vi "AlliGator Load Phasor Ratio References.vi"(8 "Error In":errorcluster, 11 "Reference File Path (default: Dialog)":path) -> (0 "Error Out":errorcluster, 1 "Reference 2 Loaded":bool, 2 "Reference 1 Loaded":bool, 3 "Phasor References":T2, 4 "Message":string)   [LabVIEW 2021, in "AlliGator Phasor Ratio.lvlib"]
doc: "Dialog to select one or both references to load."
uses:
  AlliGator Phasor Ratio.lvlib
  Phasor/Phasor (g, s).ctl
  Phasor Graph/AlliGator Phasor Ratio Reference & Lifetime v1.ctl
  AlliGator Phasor Ratio Reference & Lifetime v2.ctl
  aa7095b5-11c0-4eb5-8147-98e7219ba57f.vi
  aa7095b5-11c0-4eb5-8147-98e7219ba57f.vi/8a80743f-1319-44c8-96b0-3ef8fc688731.vi
  aa7095b5-11c0-4eb5-8147-98e7219ba57f.vi/931f4f8f-d8c6-4056-833f-5c8fe97b24b9.vi
  <vilib>/Utility/error.llb/Error Cluster From Error Code.vi
  <vilib>/ErrorRing/Error Ring.xnode
  Phasor/Phasor.lvlib
  Phasor Graph/AlliGator Phasor Graph.lvlib
  Files/Files.lvlib
  Settings/AlliGator Settings.lvlib
panel:
  in  "Cancel":bool
  in  "Load":bool
  in  "Load Reference 2":bool
  in  "Load Reference 1":bool
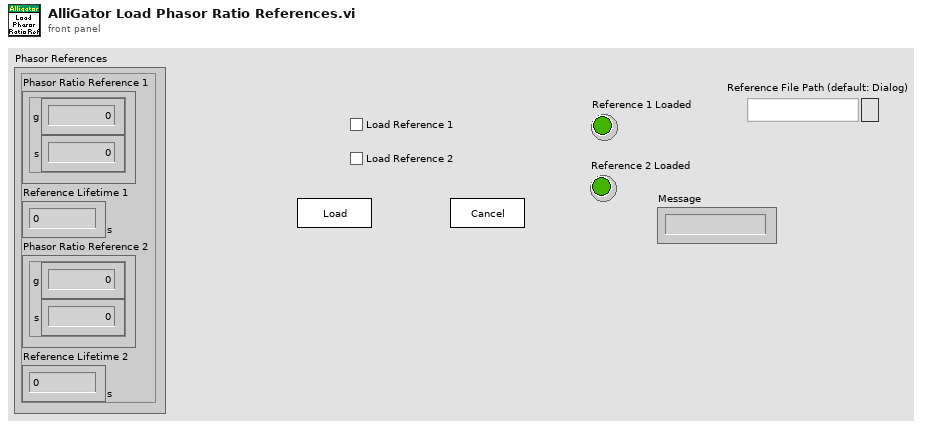
[diagram p1: front panel]
types:
  T1 = typedef "Phasor.lvlib/Phasor (g, s).ctl" = cluster{"g":dbl, "s":dbl}
  T2 = cluster{"Phasor Ratio Reference 1":T1, "Reference Lifetime 1":dbl[unit], "Phasor Ratio Reference 2":T1, "Reference Lifetime 2":dbl[unit]}
  T3 = typedef "AlliGator Phasor Ratio.lvlib/AlliGator Phasor Ratio Reference & Lifetime v2.ctl" = cluster{"Phasor Ratio Reference":T1, "Reference Lifetime":dbl[unit], "Phasor Frequency":dbl[unit]}
  T4 = typedef "AlliGator Phasor Graph.lvlib/AlliGator Phasor Ratio Reference & Lifetime v1.ctl" = cluster{"Phasor Ratio Reference 1":T1, "Reference Lifetime 1":dbl[unit]}
  T5 = enum32{"Invalid", "Standard", "Closed", "Hidden", "Minimized", "Maximized"}
  T6 = enum8{"Enabled", "Disabled", "Disabled and Grayed Out"}
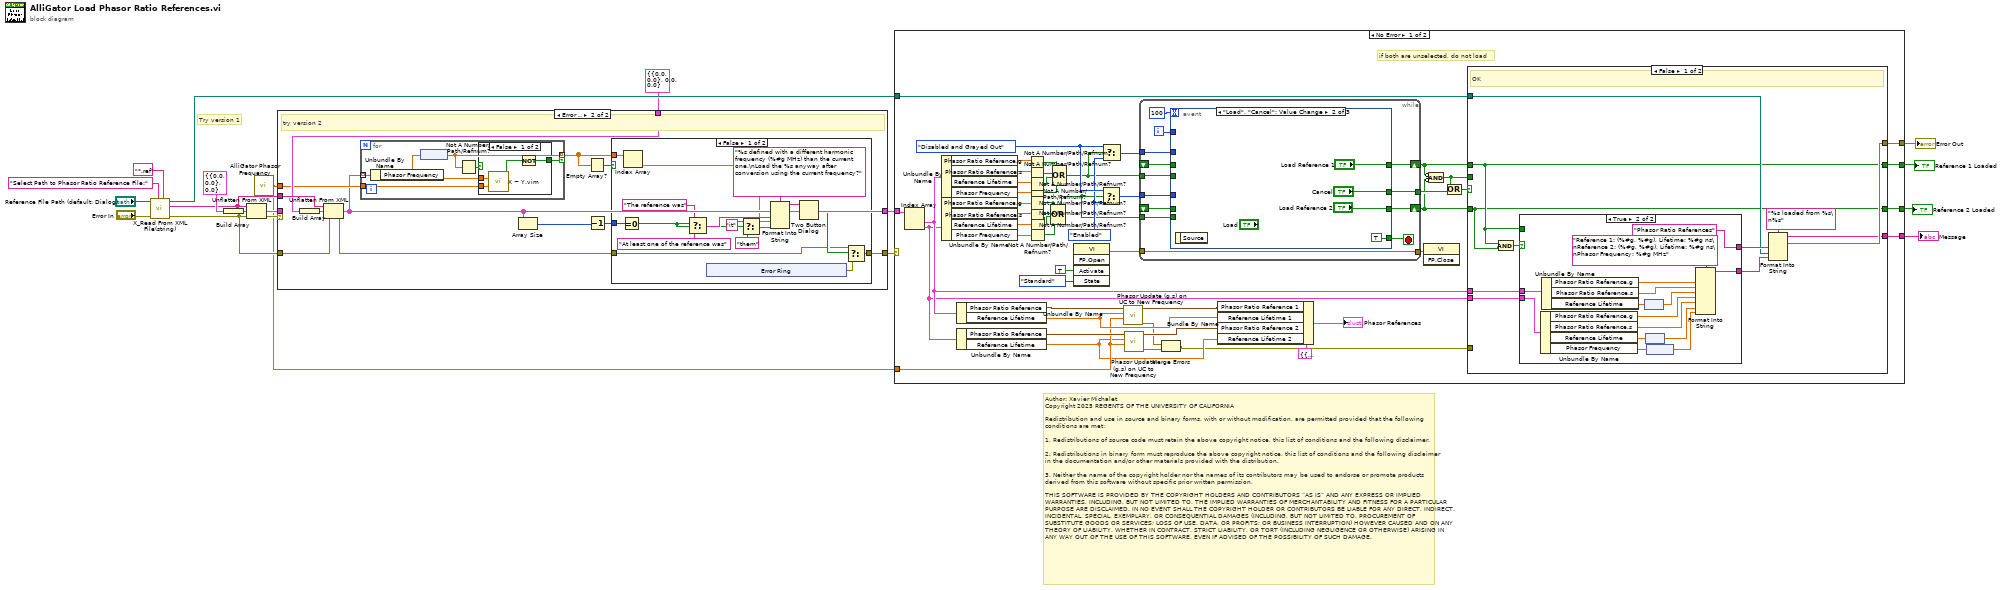
[diagram p0: block diagram]
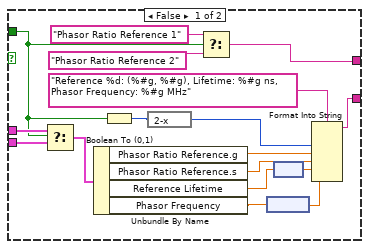
[diagram p2: hidden frame]
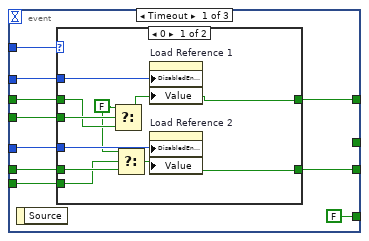
[diagram p4: hidden frame]
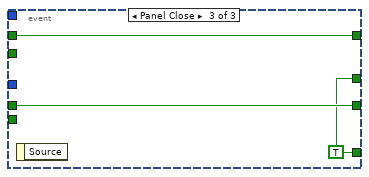
[diagram p6: hidden frame]
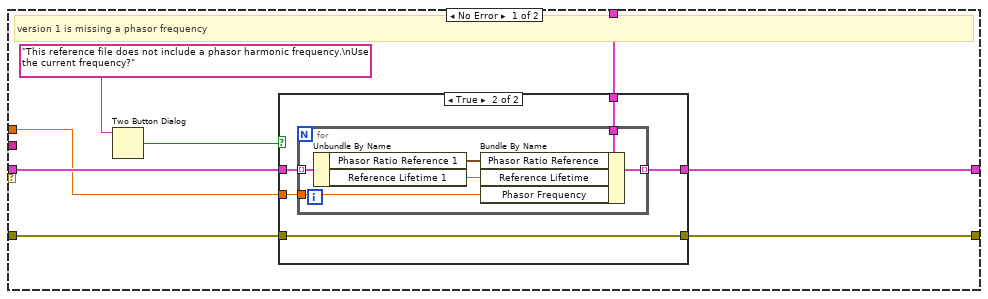
[diagram p8: hidden frame]
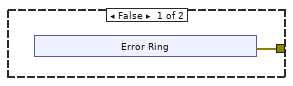
[diagram p9: hidden frame]
diagram:
  # "Author: Xavier Michalet\nCopyright 2025 REGENTS OF THE UNIVERSITY OF CALIFORNIA\n\nRedistribution and use in source and binary forms, with or without modification, are permitted provided that the following conditions are met:\n\n1. Redistributions of source code must retain the above copyright notice, this list of conditions and the following disclaimer.\n\n2. Redistributions in binary form must reproduce the above copyright notice, this list of conditions and the following disclaimer in the documentation and/or other materials provided with the distribution.\n\n3. Neither the name of the copyright holder nor the names of its contributors may be used to endorse or promote products derived from this software without specific prior written permission.\n\nTHIS SOFTWARE IS PROVIDED BY THE COPYRIGHT HOLDERS AND CONTRIBUTORS “AS IS” AND ANY EXPRESS OR IMPLIED WARRANTIES, INCLUDING, BUT NOT LIMITED TO, THE IMPLIED WARRANTIES OF MERCHANTABILITY AND FITNESS FOR A PARTICULAR PURPOSE ARE DISCLAIMED. IN NO EVENT SHALL THE COPYRIGHT HOLDER OR CONTRIBUTORS BE LIABLE FOR ANY DIRECT, INDIRECT, INCIDENTAL, SPECIAL, EXEMPLARY, OR CONSEQUENTIAL DAMAGES (INCLUDING, BUT NOT LIMITED TO, PROCUREMENT OF SUBSTITUTE GOODS OR SERVICES; LOSS OF USE, DATA, OR PROFITS; OR BUSINESS INTERRUPTION) HOWEVER CAUSED AND ON ANY THEORY OF LIABILITY, WHETHER IN CONTRACT, STRICT LIABILITY, OR TORT (INCLUDING NEGLIGENCE OR OTHERWISE) ARISING IN ANY WAY OUT OF THE USE OF THIS SOFTWARE, EVEN IF ADVISED OF THE POSSIBILITY OF SUCH DAMAGE."
  # "Try version 1"
  n1 = call "X_Read From XML File(string).vi"("pattern (*.xml)"="*.ref", "Prompt"="Select Path to Phasor Ratio Reference File:", "error in (no error)"="Error In", "XML File Path"="Reference File Path (default: Dialog)") -> ("error out"=w12:errorcluster, "XML Elements"=w11:string, "XML File Path(duplicate)"=w16:path)  [unwired: 5 in]
  n2 = Build Array(T4 {"Phasor Ratio Reference 1"={"g"=0.0, "s"=0.0}, "Reference Lifetime 1"=0.0} ("appended array")) -> (w7:T4[])
  n3 = Unflatten From XML(xml string=w11, type=w7, error in (no error)=w12) -> (value=w8:T4[], error out=w13:errorcluster)
  n4 = call "AlliGator Phasor Frequency.vi"() -> ("Phasor Frequency"=w1:dbl[unit])
  n5 = case shown="Error .." w13 {
    tunnel: w12 -> [w22 w55]
    tunnel: w11 -> [_ w54]
    tunnel: [w21 w49] -> w6
    tunnel: [w25 w48] -> w10
    tunnel: T3 {"Phasor Ratio Reference"={"g"=0.0, "s"=0.0}, "Reference Lifetime"=0.0, "Phasor Frequency"=0.0} ("appended array") -> [w26 w53]
    tunnel: w8 -> [w27 _]
    tunnel: w1 -> [w20 w51]
    frame No Error {
      # "version 1 is missing a phasor frequency"
      n6 = Two Button Dialog(message="This reference file does not include a phasor harmonic frequency.\nUse the current frequency?") -> (T button?=w23:bool)  [unwired: 2 in]
      n7 = case shown="True" w23 {
        tunnel: w27 -> [_ w37]
        tunnel: w26 -> [_ w36]
        tunnel: [_ w35] -> w25
        tunnel: w22 -> [_ w34]
        tunnel: [w28 w34] -> w21
        tunnel: w20 -> [_ w33]
        frame False {
          n8 = xnode "Error Ring"() -> ("error out"=w28:errorcluster)
        }
        frame True {
          n9 = for {
            tunnel: w37 -> [w43] mode=indexing
            tunnel: w36 -> [w42]
            tunnel: [w39] -> w35 mode=indexing
            tunnel: w33 -> [w38]
            n10 = Unbundle By Name(w43) -> ("Phasor Ratio Reference 1"=w41:T1, "Reference Lifetime 1"=w40:dbl[unit])
            n11 = Bundle By Name(cluster=w42, "Phasor Ratio Reference"=w41, "Reference Lifetime"=w40, "Phasor Frequency"=w38) -> (w39:T3)
          }
        }
      }
    }
    frame Error {
      # "try version 2"
      n12 = Build Array(w53) -> (w52:T3[])
      n13 = Unflatten From XML(xml string=w54, type=w52, error in (no error)=w55) -> (value=w48:T3[], error out=w50:errorcluster)
      n14 = for {
        tunnel: w48 -> [w82] mode=indexing
        tunnel: w51 -> [w81]
        tunnel: [w78] -> w45 mode=indexing if=w80
        n15 = Unbundle By Name(w82) -> ("Phasor Frequency"=w79:dbl[unit])
        n16 = node(w79) -> (w78:dbl)
        n17 = Not A Number/Path/Refnum?(number/path/refnum=w78) -> (NaN/Path/Refnum?=w77:bool)
        n18 = case shown="False" w77 {
          tunnel: w81 -> [w86 _]
          tunnel: [w84 _] -> w80
          tunnel: w79 -> [w83 _]
          frame False {
            n19 = call "X ~ Y.vim"("X"=w83, "Y"=w86) -> ("X ~= Y?"=w85:bool)  [unwired: 13 in]
            n20 = Not(x=w85) -> (.not. x?=w84:bool)
          }
          frame True {
          }
        }
      }
      n21 = Array Size(array=w48) -> (size(s)=w47:i32)
      n22 = Empty Array?(array=w45) -> (empty?=w44:bool)
      n23 = Decrement(x=w47) -> (x-1=w46:i32)
      n24 = case shown="False" w44 {
        tunnel: w50 -> [w58 w76]
        tunnel: [w59 w76] -> w49
        tunnel: w46 -> [w69 _]
        tunnel: w45 -> [w57 _]
        frame False {
          n25 = Equal To 0?(x=w69) -> (x = 0?=w65:bool)
          n26 = Index Array(array=w57) -> (element=w56:dbl)  [unwired: 1 in]
          n27 = Select(t="The reference was" ("message"), s=w65, f="At least one of the reference was" ("message")) -> (s? t:f=w66:string)
          n28 = xnode "Error Ring"() -> ("error out"=w60:errorcluster)
          n29 = Select(t="it" ("message"), s=w65, f="them" ("message")) -> (s? t:f=w62:string)
          n30 = Format Into String(format string="%s defined with a different harmonic frequency (%#g MHz) than the current one.\nLoad the %s anyway after conversion using the current frequency?", w66, w56, w62) -> (resulting string=w71:string)  [unwired: 2 in, 1 out]
          n31 = Two Button Dialog(message=w71) -> (T button?=w61:bool)  [unwired: 2 in]
          n32 = Select(t=w58, s=w61, f=w60) -> (s? t:f=w59:errorcluster)
        }
        frame True {
        }
      }
    }
  }
  n33 = case shown="No Error" w6 {
    selector: w6 -> [_ w222]
    tunnel: [w137 w222] -> w19
    tunnel: w16 -> [w136 _]
    tunnel: [w135 _] -> w15
    tunnel: [w134 _] -> w14
    tunnel: w10 -> [w105 _]
    tunnel: [w99 _] -> w5
    tunnel: w1 -> [w91 _]
    frame No Error {
      w132 = T6."Enabled" ("Disabled")
      w133 = T6."Disabled and Grayed Out" ("Disabled")
      # "if both are unselected, do not load"
      n34 = Index Array(array=w105) -> (element #1=w98:T3, element #2=w97:T3)  [unwired: 2 in]
      n35 = Unbundle By Name(w98) -> ("Phasor Ratio Reference.g"=w116:dbl, "Phasor Ratio Reference.s"=w115:dbl, "Reference Lifetime"=w114:dbl[unit], "Phasor Frequency"=w102:dbl[unit])
      n36 = Unbundle By Name(w97) -> ("Phasor Ratio Reference.g"=w113:dbl, "Phasor Ratio Reference.s"=w112:dbl, "Reference Lifetime"=w111:dbl[unit], "Phasor Frequency"=w104:dbl[unit])
      n37 = Unbundle By Name(w98) -> ("Phasor Ratio Reference"=w96:T1, "Reference Lifetime"=w94:dbl[unit])
      n38 = Unbundle By Name(w97) -> ("Phasor Ratio Reference"=w93:T1, "Reference Lifetime"=w90:dbl[unit])
      n39 = Not A Number/Path/Refnum?(number/path/refnum=w116) -> (NaN/Path/Refnum?=w122:bool)
      n40 = Not A Number/Path/Refnum?(number/path/refnum=w115) -> (NaN/Path/Refnum?=w124:bool)
      n41 = Not A Number/Path/Refnum?(number/path/refnum=w114) -> (NaN/Path/Refnum?=w123:bool)
      n42 = Not A Number/Path/Refnum?(number/path/refnum=w102) -> (NaN/Path/Refnum?=w101:bool)
      n43 = Not A Number/Path/Refnum?(number/path/refnum=w113) -> (NaN/Path/Refnum?=w119:bool)
      n44 = Not A Number/Path/Refnum?(number/path/refnum=w112) -> (NaN/Path/Refnum?=w120:bool)
      n45 = Not A Number/Path/Refnum?(number/path/refnum=w111) -> (NaN/Path/Refnum?=w118:bool)
      n46 = Not A Number/Path/Refnum?(number/path/refnum=w104) -> (NaN/Path/Refnum?=w103:bool)
      n47 = Compound Arithmetic op=OR(w119, w120, w118, w103) -> (w117:bool)
      n48 = Compound Arithmetic op=OR(w122, w124, w123, w101) -> (w121:bool)
      n49 = invoke class="VI" method="FP.Open"("Activate"=TRUE ("Activate?"), "State"=T5."Standard") -> (error out=w106:errorcluster)  [unwired: 3 in, 4 out]
      n50 = Select(t=w133, s=w117, f=w132) -> (s? t:f=w130:T6)
      n51 = Select(t=w133, s=w121, f=w132) -> (s? t:f=w131:T6)
      n52 = call "Phasor Update (g,s) on UC to New Frequency.vi"("New Phasor Frequency"=w91, "Lifetime"=w94, "Phasor in"=w96) -> ("Error Out"=w88:errorcluster, "Phasor out"=w95:T1)  [unwired: 7 in]
      n53 = call "Phasor Update (g,s) on UC to New Frequency.vi"("New Phasor Frequency"=w91, "Lifetime"=w90, "Phasor in"=w93) -> ("Error Out"=w89:errorcluster, "Phasor out"=w92:T1)  [unwired: 7 in]
      n54 = while {
        tunnel: w131 -> [w193]
        tunnel: w130 -> [w192]
        shift-right: [w187] -> w127
        shift-left: _ -> [w190]
        tunnel: w121 -> [w191]
        shift-right: [w186] -> w126
        shift-left: _ -> [w184]
        tunnel: w117 -> [w185]
        tunnel: [w182] -> w129
        tunnel: w106 -> [w181]
        tunnel: [w181] -> w100
        i -> [w188]
        stop <- w183 stop-if-true
        n55 = event shown="[1] \"Load\", \"Cancel\": Value Change" {
          selector: _ -> [_ _ _]
          dyn-events: _ -> [_ _ _]
          timeout: 100 -> [_ _ _]
          tunnel: w193 -> [w203 _ _]
          tunnel: w192 -> [w202 _ _]
          tunnel: w191 -> [w201 _ _]
          tunnel: w190 -> [w200 _ w221]
          tunnel: w188 -> [w199 _ _]
          tunnel: [w198 "Load Reference 1" w221] -> w187
          tunnel: [w197 "Load Reference 2" w220] -> w186
          tunnel: w185 -> [w195 _ _]
          tunnel: w184 -> [w196 _ w220]
          tunnel: [FALSE TRUE w219] -> w183
          tunnel: [_ "Cancel" w219] -> w182
          event Timeout {
            n56 = event-data() -> ()  [unwired: 1 in, 1 out]
            n57 = case shown="0" w199 {
              tunnel: w203 -> [w212 _]
              tunnel: w202 -> [w211 _]
              tunnel: w201 -> [w210 _]
              tunnel: w200 -> [w209 w214]
              tunnel: [w208 w214] -> w198
              tunnel: [w204 w213] -> w197
              tunnel: w196 -> [w206 w213]
              tunnel: w195 -> [w205 _]
              frame 0 {
                w207 = FALSE
                n58 = Select(t=w207, s=w210, f=w209) -> (s? t:f=w208:bool)
                n59 = Select(t=w207, s=w205, f=w206) -> (s? t:f=w204:bool)
                n60 = property on="Load Reference 1" class="Bool (strict)"("DisabledEnum"=w212, "Value"=w208) -> ()  [unwired: 2 in, 2 out]
                n61 = property on="Load Reference 2" class="Bool (strict)"("DisabledEnum"=w211, "Value"=w204) -> ()  [unwired: 2 in, 2 out]
              }
              frame 1, Default {
              }
            }
          }
          event "Load", "Cancel": Value Change {
            n62 = event-data() -> ()  [unwired: 1 in, 1 out]
          }
          event Panel Close {
            w219 = TRUE
            n63 = event-data() -> ()  [unwired: 1 in, 1 out]
          }
        }
      }
      n64 = Merge Errors(w88, w89) -> (w87:errorcluster)
      n65 = Bundle By Name(cluster=T2 {"Phasor Ratio Reference 1"={"g"=0.0, "s"=0.0}, "Reference Lifetime 1"=0.0, "Phasor Ratio Reference 2"={"g"=0.0, "s"=0.0}, "Reference Lifetime 2"=0.0} ("Phasor References"), "Phasor Ratio Reference 1"=w95, "Reference Lifetime 1"=w94, "Phasor Ratio Reference 2"=w92, "Reference Lifetime 2"=w90) -> (→"Phasor References":T2)
      n66 = invoke class="VI" method="FP.Close"(error in=w100) -> ()  [unwired: 2 in, 3 out]
      n67 = Compound Arithmetic op=AND(invert w127, invert w126) -> (w125:bool)
      n68 = Compound Arithmetic op=OR(w125, w129) -> (w128:bool)
      n69 = case shown="False" w128 {
        tunnel: [w145 _] -> w137
        tunnel: w127 -> [w143 _]
        tunnel: w126 -> [w142 _]
        tunnel: w125 -> [_ _]
        tunnel: w136 -> [w144 _]
        tunnel: [w143 _] -> w135
        tunnel: [w142 _] -> w134
        tunnel: [w141 _] -> w99
        tunnel: w98 -> [w140 _]
        tunnel: w97 -> [w139 _]
        tunnel: w87 -> [_ _]
        frame False {
          # "OK"
          n70 = And(x=w143, y=w142) -> (x .and. y?=w148:bool)
          n71 = case shown="True" w148 {
            tunnel: [w163 "Phasor Ratio References" ("format string")] -> w147
            tunnel: w143 -> [w155 _]
            tunnel: w140 -> [w162 w177]
            tunnel: w139 -> [w161 w176]
            tunnel: [w152 w168] -> w138
            frame False {
              n72 = Select(t=w162, s=w155, f=w161) -> (s? t:f=w160:T3)
              n73 = Unbundle By Name(w160) -> ("Phasor Ratio Reference.g"=w158:dbl, "Phasor Ratio Reference.s"=w157:dbl, "Reference Lifetime"=w156:dbl[unit], "Phasor Frequency"=w150:dbl[unit])
              n74 = Boolean To (0,1)(Boolean=w155) -> (0, 1=w154:i16)
              n75 = expression code="2-x"(w154) -> (w153:i16)
              n76 = Select(t="Phasor Ratio Reference 1" ("format string"), s=w155, f="Phasor Ratio Reference 2" ("format string")) -> (s? t:f=w163:string)
              n77 = node(w150) -> (w149:dbl)
              n78 = node(w156) -> (w151:dbl)
              n79 = Format Into String(format string="Reference %d: (%#g, %#g), Lifetime: %#g ns, Phasor Frequency: %#g MHz", w153, w158, w157, w151, w149) -> (resulting string=w152:string)  [unwired: 2 in, 1 out]
            }
            frame True {
              n80 = Unbundle By Name(w176) -> ("Phasor Ratio Reference.g"=w171:dbl, "Phasor Ratio Reference.s"=w170:dbl, "Reference Lifetime"=w178:dbl[unit], "Phasor Frequency"=w167:dbl[unit])
              n81 = Unbundle By Name(w177) -> ("Phasor Ratio Reference.g"=w174:dbl, "Phasor Ratio Reference.s"=w173:dbl, "Reference Lifetime"=w179:dbl[unit])
              n82 = node(w179) -> (w172:dbl)
              n83 = node(w178) -> (w169:dbl)
              n84 = node(w167) -> (w166:dbl)
              n85 = Format Into String(format string="Reference 1: (%#g, %#g), Lifetime: %#g ns\nReference 2: (%#g, %#g), Lifetime: %#g ns\nPhasor Frequency: %#g MHz", w174, w173, w172, w171, w170, w169, w166) -> (resulting string=w168:string)  [unwired: 2 in, 1 out]
            }
          }
          n86 = Format Into String(format string="%s loaded from %s\n%s", w147, w144, w138) -> (resulting string=w141:string, error out=w145:errorcluster)  [unwired: 2 in]
        }
        frame True {
          # "Cancelled"
        }
      }
    }
    frame Error {
    }
  }
  "Error Out" <- w19
  "Reference 1 Loaded" <- w15
  "Reference 2 Loaded" <- w14
  "Message" <- w5
